vi "Parse Response.vi"(8 "error in (no error)":errorcluster, 10 "{JSON} Response":string, 11 "JSON-RPC in":refnum<class "JSON-RPC.lvclass">) -> (0 "error out":errorcluster, 1 "Equal?":bool, 2 "results":string, 3 "JSON-RPC out":refnum<class "JSON-RPC.lvclass">, 4 "IDs":string)   [LabVIEW 2019, in "JSON-RPC.lvclass"]
uses:
  JSON-RPC.lvclass
  JSON-RPC.lvclass/JSON-RPC.ctl
  private/Parse Response-JSONtext.vi/7ce7fba8-9f44-478d-b6cb-b571ff29f2f5.vi
  private/Parse Response-JSONtext.vi/8c905beb-ab4c-49e3-b5c6-2c663b7b30d7.vi
  private/Parse Response-JSONtext.vi/fce5892e-0c40-47e1-88e0-6c122aadefe2.vi
  <vilib>/JDP Science/JSONtext/Find Item.vi
  <vilib>/JDP Science/JSONtext/Next JSON Value.vi
  <vilib>/JDP Science/JSONtext/String Subset.vi
  <vilib>/JDP Science/JSONtext/Parsing/Advance past next JSON Value (inlined COPY).vi
  <vilib>/JDP Science/JSONtext/Parsing/Advance past whitespace.vi
  <vilib>/JDP Science/JSONtext/Parsing/Advance past String.vi
  <vilib>/JDP Science/JSONtext/Parsing/Advance past Number.vi
  <vilib>/JDP Science/JSONtext/Parsing/Advance past Line Ending.vi
  <vilib>/JDP Science/JSONtext/Get all Object Items.vi
  <vilib>/JDP Science/JSONtext/Parsing/Parse Full Path or Item Name.vi
  <vilib>/JDP Science/JSONtext/Parsing/Advance past Array.vi
  <vilib>/JDP Science/JSONtext/Parsing/Advance past Object.vi
  <vilib>/JDP Science/JSONtext/support/Error Cluster From Code.vi
  <vilib>/JDP Science/JSONtext/Offset/Find Item Locations by Path.vi
  <vilib>/JDP Science/JSONtext/JSON text to Variant.vi
  <vilib>/Utility/error.llb/Error Cluster From Error Code.vi
  <vilib>/JDP Science/JSONtext/LVClass Serializer/JSONtext LVClass Serializer.lvclass
  <vilib>/JDP Science/JSONtext/JSONtext.lvlib
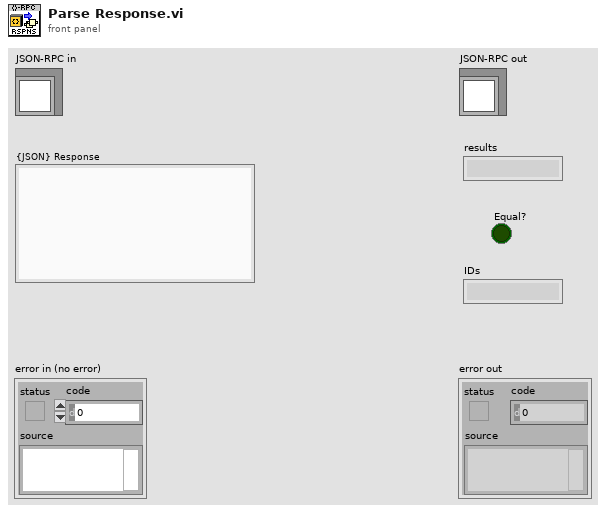
[diagram p1: front panel]
types:
  T1 = typedef "JSONtext.lvlib/JSON Value Type.ctl" = enum16{"Not a JSON Value", "JSON Object", "JSON Array", "String", "Number", "true", "false", "null"}
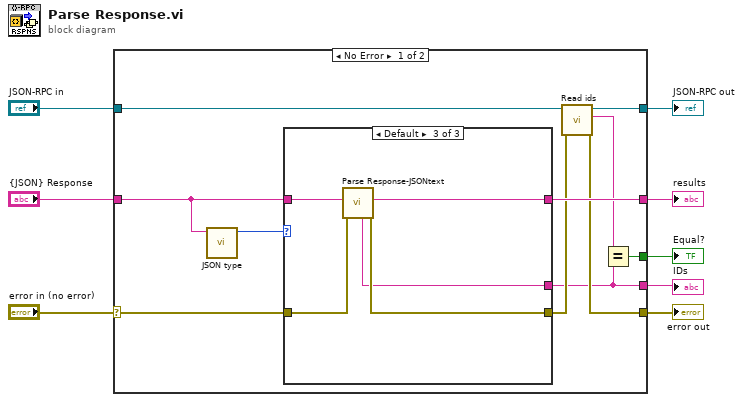
[diagram p0: block diagram]
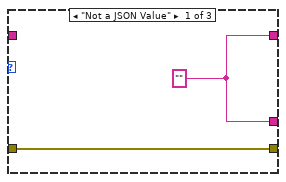
[diagram p2: hidden frame]
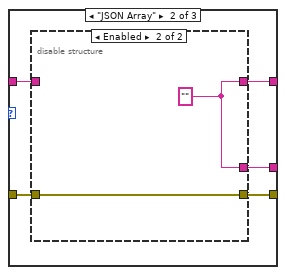
[diagram p3: hidden frame]
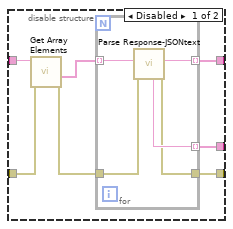
[diagram p4: hidden frame]
diagram:
  n1 = case shown="No Error" "error in (no error)" {
    selector: "error in (no error)" -> [w17 w47]
    tunnel: [w12 w47] -> w7
    tunnel: "JSON-RPC in" -> [w14 w46]
    tunnel: "{JSON} Response" -> [w18 _]
    tunnel: [w15 w46] -> w4
    tunnel: [w16 _] -> w3
    tunnel: [w10 _] -> w2
    tunnel: [w9 _] -> w1
    frame No Error {
      n2 = call <vilib>:"JSON type.vi"("JSON"=w18) -> ("JSON Value Type"=w19:T1)  [unwired: 9 in, 1 out]
      n3 = case shown="Default" w19 {
        tunnel: w17 -> [w21 w23 w44]
        tunnel: [w21 w26 w43] -> w13
        tunnel: w18 -> [_ w24 w45]
        tunnel: [w20 w25 w41] -> w16
        tunnel: [w20 w22 w42] -> w9
        frame "Not a JSON Value" {
          w20 = ""
        }
        frame "JSON Array" {
          n4 = disable-structure shown="Enabled" {
            disable-tunnel: [w33 w39] -> w26
            disable-tunnel: [w32 w40] -> w25
            disable-tunnel: w24 -> [w31 _]
            disable-tunnel: w23 -> [w30 w39]
            disable-tunnel: [w28 w40] -> w22
            frame Disabled {
              n5 = call <vilib>:"Get Array Elements.vi"("error in (no error)"=w30, "JSON"=w31) -> ("error out"=w27:errorcluster, "<JSON>"=w29:string[])  [unwired: 7 in, 1 out]
              n6 = for {
                tunnel: w29 -> [w38] mode=indexing
                tunnel: [w36] -> w32 mode=indexing
                tunnel: [w35] -> w28 mode=indexing
                tunnel: w27 -> [w37]
                tunnel: [w34] -> w33
                n7 = call "Parse Response-JSONtext.vi"("error in (no error)"=w37, "{JSON} Response"=w38) -> ("error out"=w34:errorcluster, "result"=w36:string, "id"=w35:string)  [unwired: 7 in]
              }
            }
            frame Enabled {
              w40 = ""
            }
          }
        }
        frame Default {
          n8 = call "Parse Response-JSONtext.vi"("error in (no error)"=w44, "{JSON} Response"=w45) -> ("error out"=w43:errorcluster, "result"=w41:string, "id"=w42:string)  [unwired: 7 in]
        }
      }
      n9 = call "Read ids.vi"("error in (no error)"=w13, "JSON-RPC in"=w14) -> ("error out"=w12:errorcluster, "ids"=w11:string, "JSON-RPC out"=w15:refnum<class "JSON-RPC.lvclass">)  [unwired: 7 in]
      n10 = Equal?(x=w11, y=w9) -> (x = y?=w10:bool)
    }
    frame Error {
    }
  }
  "error out" <- w7
  "JSON-RPC out" <- w4
  "results" <- w3
  "Equal?" <- w2
  "IDs" <- w1
